vi "controlArray_to_JSON.vi"(8 "error in":errorcluster, 10 "refDesArray":string[](array[string]), 11 "Control Data Type":dbl[](array[numeric])) -> (0 "error out":errorcluster, 3 "Data JSON":string)   [LabVIEW 2024]
uses:
  Control/webSocketJsonData.ctl
panel:
  in  "webSocketJsonData":T1={"type"="data", "t"=0.0, "d"=[{"r"="", "v"=0.0}]}
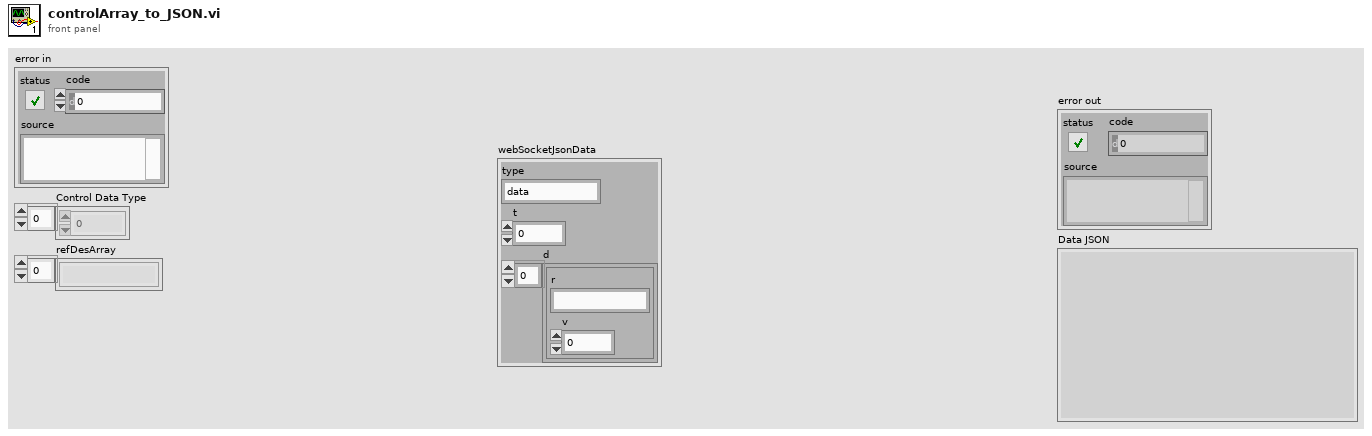
[diagram p1: front panel]
types:
  T1 = typedef "webSocketJsonData.ctl" = cluster{"type":string, "t":dbl, "d":cluster{"r":string, "v":dbl}[]}
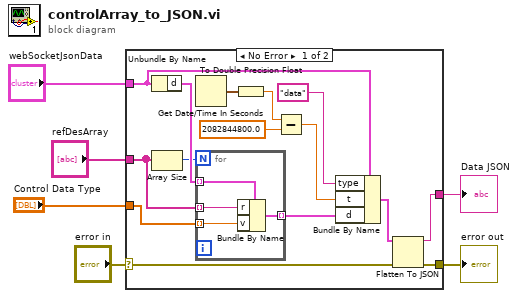
[diagram p0: block diagram]
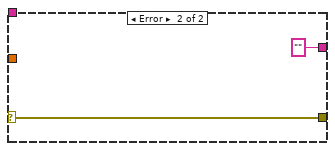
[diagram p2: hidden frame]
diagram:
  n1 = case shown="No Error" "error in" {
    selector: "error in" -> [w21 w27]
    tunnel: [w20 w27] -> w5
    tunnel: [w19 "" ("JSON string")] -> w4
    tunnel: "Control Data Type" -> [w9 _]
    tunnel: "webSocketJsonData" -> [w12 _]
    tunnel: "refDesArray" -> [w7 _]
    frame No Error {
      n2 = Unbundle By Name(w12) -> ("d"=w11:cluster{"r":string, "v":dbl}[])
      n3 = Array Size(array=w7) -> (size(s)=w10:i32)
      n4 = Get Date/Time In Seconds() -> (seconds since 1Jan1904=w16:timestamp)
      n5 = for {
        N: w10 -> [_]
        tunnel: w11 -> [w25] mode=indexing
        tunnel: w9 -> [w24] mode=indexing
        tunnel: [w23] -> w8 mode=indexing
        tunnel: w7 -> [w22] mode=indexing
        n6 = Bundle By Name(cluster=w25, "r"=w22, "v"=w24) -> (w23:cluster{"r":string, "v":dbl})
      }
      n7 = To Double Precision Float(number=w16) -> (double precision float=w15:dbl)
      n8 = Subtract(x=w15, y=2082844800.0) -> (x-y=w13:dbl)
      n9 = Bundle By Name(cluster=w12, "type"="data", "t"=w13, "d"=w8) -> (w18:T1)
      n10 = Flatten To JSON(anything=w18, error in (no error)=w21) -> (JSON string=w19:string, 11:w20:errorcluster)  [unwired: 1 in]
    }
    frame Error {
    }
  }
  "error out" <- w5
  "Data JSON" <- w4
